vi "Database Queue Handler.vi"(7 "Action":T3, 8 "error in (no error)":errorcluster, 10 "Message in":T1, 11 "Queue in":refnum<queue>) -> (0 "error out":errorcluster, 2 "Message out":T1, 3 "Queue out":refnum<queue>)   [LabVIEW 2017]
uses:
  Type Definitions/Queue FG Options.ctl
  Type Definitions/Database Message.ctl
  Type Definitions/Database States.ctl
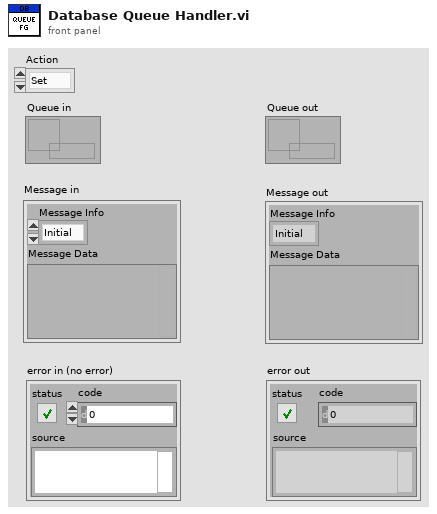
[diagram p1: front panel]
types:
  T1 = typedef "Database Message.ctl" = cluster{"Message Info":T2, "Message Data":variant}
  T2 = typedef "Database States.ctl" = enum16{"Initial", "Verify", "Balance Inquiry", "Deposit", "Withdrawal", "Fast Cash", "Terminate", "Shutdown"}
  T3 = typedef "Queue FG Options.ctl" = enum16{"Set", "Get", "Read", "Write", "Destroy"}
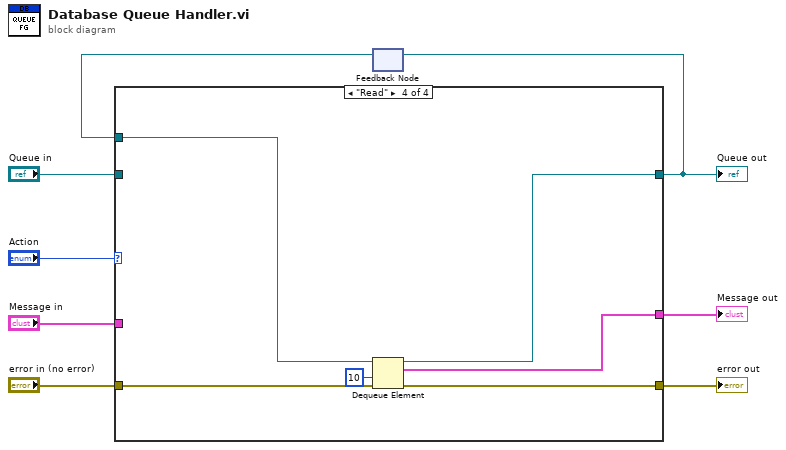
[diagram p0: block diagram]
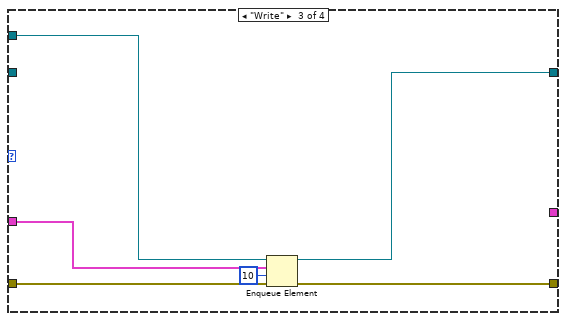
[diagram p4: hidden frame]
diagram:
  n1 = feedback #1() -> (w5:refnum<queue>)  [unwired: 1 in]
  n2 = case shown="\"Read\"" "Action" {
    tunnel: "error in (no error)" -> [w10 w12 w18 w24]
    tunnel: [w10 w12 w17 w23] -> w6
    tunnel: w5 -> [_ w11 w16 w22]
    tunnel: "Message in" -> [_ _ w15 _]
    tunnel: [w9 w11 w14 w21] -> w3
    tunnel: "Queue in" -> [w9 _ _ _]
    tunnel: [_ _ _ w20] -> w1
    frame "Set" {
    }
    frame "Get", Default {
    }
    frame "Write" {
      n3 = Enqueue Element(queue=w16, element=w15, timeout in ms (-1)=10, error in (no error)=w18) -> (queue out=w14:refnum<queue>, error out=w17:errorcluster)  [unwired: 1 out]
    }
    frame "Read" {
      n4 = Dequeue Element(queue=w22, timeout in ms (-1)=10, error in (no error)=w24) -> (queue out=w21:refnum<queue>, element=w20:T1, error out=w23:errorcluster)  [unwired: 1 out]
    }
  }
  "error out" <- w6
  "Message out" <- w1
  "Queue out" <- w3
  n5 = feedback-in #1(w3) -> ()
